vi "replaceSpaceWithHyphen.vi"(10 "stringIn":string) -> (2 "stringOut":string)   [LabVIEW 2020]
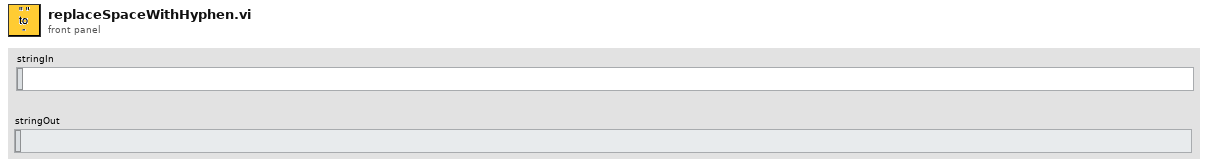
[diagram p1: front panel]
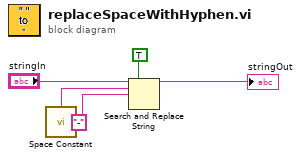
[diagram p0: block diagram]
diagram:
  n1 = call <vilib>:"Space Constant.vi"() -> ("String"=w4:string)
  n2 = Search and Replace String(replace all?=TRUE ("replace all? (F)"), input string="stringIn", search string=w4, replace string="-" ("replace string (\"\")")) -> (result string=→"stringOut":string)  [unwired: 4 in, 3 out]
